vi "Free.vi"(8 "error in (no error)":errorcluster, 11 "MsgPackDeserializer.lvclass":refnum<class "MsgPackDeserializer.lvclass">) -> (0 "error IO":errorcluster, 3 "rest":string)   [LabVIEW 2015, in "MsgPackDeserializer.lvclass"]
uses:
  MsgPackDeserializer.lvclass
  MsgPackDeserializer.lvclass/MsgPackDeserializer.ctl
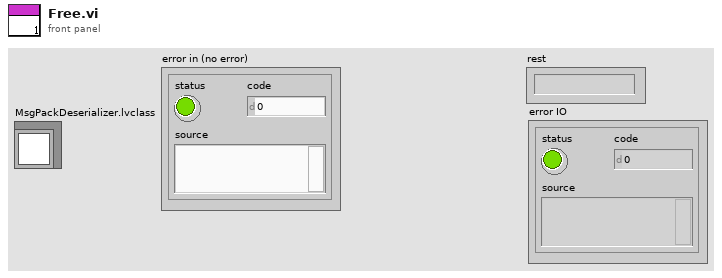
[diagram p1: front panel]
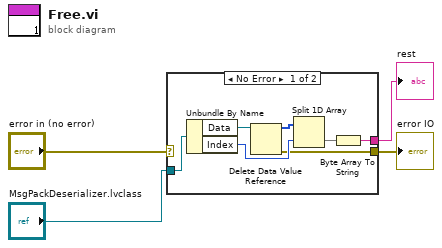
[diagram p0: block diagram]
diagram:
  n1 = case shown="No Error" "error in (no error)" {
    selector: "error in (no error)" -> [_ w12]
    tunnel: "MsgPackDeserializer.lvclass" -> [w9 _]
    tunnel: [w6 _] -> w3
    tunnel: [w5 w12] -> w2
    frame No Error {
      n2 = Unbundle By Name(w9) -> ("Data"=w11:refnum<data-value>, "Index"=w8:i64)
      n3 = Delete Data Value Reference(data value reference=w11) -> (data value=w10:u8[], error out=w5:errorcluster)  [unwired: 1 in]
      n4 = Split 1D Array(array=w10, index=w8) -> (second subarray=w7:u8[])  [unwired: 1 out]
      n5 = Byte Array To String(unsigned byte array=w7) -> (string=w6:string)
    }
    frame Error {
    }
  }
  "rest" <- w3
  "error IO" <- w2
